vi "Write Library Ref.vi"(8 "error in (no error)":errorcluster, 10 "Library Ref":refnum<vi>, 11 "Library in":refnum<class "Library.lvclass">) -> (0 "error out":errorcluster, 3 "Library out":refnum<class "Library.lvclass">)   [LabVIEW 2019, in "Library.lvclass"]
uses:
  Library.lvclass
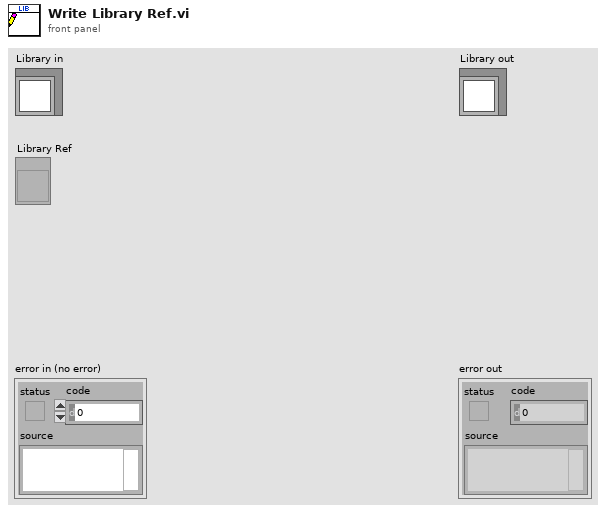
[diagram p1: front panel]
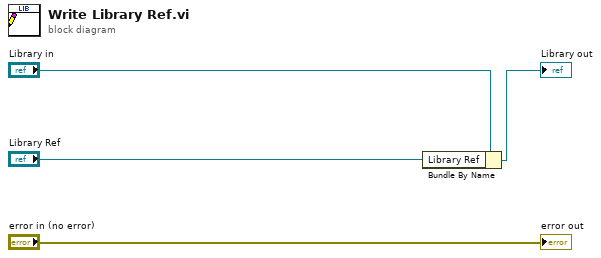
[diagram p0: block diagram]
diagram:
  n1 = Bundle By Name(cluster="Library in", "Library Ref"="Library Ref") -> (→"Library out":refnum<class "Library.lvclass">)
  "error out" <- "error in (no error)"
